vi "Check If Gif Valid.vi"(8 "error in (no error)":errorcluster caption="错误输入（无错误）", 9 "Version":string, 10 "Signature":string, 11 "Gif Image 输入":refnum<class "Gif Image.lvclass"> caption="DNL_LabVIEW Object in") -> (0 "error out":errorcluster caption="错误输出", 2 "Valid":bool, 3 "Gif Image 输出":refnum<class "Gif Image.lvclass"> caption="DNL_LabVIEW Object out")   [LabVIEW 2012, in "Picture Box Tools.lvlib" / "Gif Image.lvclass"]
uses:
  Gif Image.lvclass
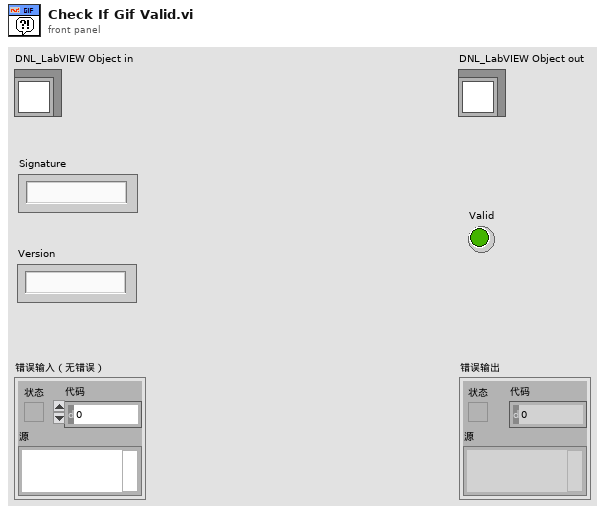
[diagram p1: front panel]
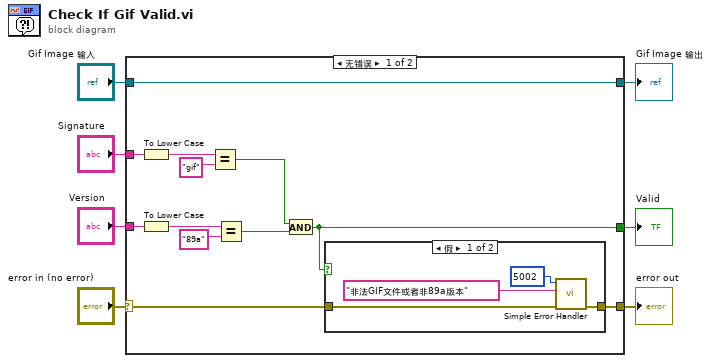
[diagram p0: block diagram]
diagram:
  n1 = case shown="无错误" "error in (no error)" {
    selector: "error in (no error)" -> [w9 w26]
    tunnel: [w8 w26] -> w6
    tunnel: [w19 w25] -> w4
    tunnel: "Gif Image 输入" -> [w19 w25]
    tunnel: "Signature" -> [w18 _]
    tunnel: "Version" -> [w17 _]
    tunnel: [w10 _] -> w1
    frame No Error {
      n2 = To Lower Case(string=w18) -> (all lower case string=w16:string)
      n3 = To Lower Case(string=w17) -> (all lower case string=w14:string)
      n4 = Equal?(x=w16, y="gif") -> (x = y?=w12:bool)
      n5 = Equal?(x=w14, y="89a") -> (x = y?=w11:bool)
      n6 = And(x=w12, y=w11) -> (x .and. y?=w10:bool)
      n7 = case shown="假" w10 {
        tunnel: w9 -> [w21 w24]
        tunnel: [w20 w24] -> w8
        frame False {
          n8 = call <vilib>:"Simple Error Handler.vi"("error code (no error:0)"=5002, "error source (\" \")"="非法GIF文件或者非89a版本" ("error source (\" \")"), "error in (no error)"=w21) -> ("error out"=w20:errorcluster)  [unwired: 2 in, 4 out]
        }
        frame True {
        }
      }
    }
    frame Error {
    }
  }
  "error out" <- w6
  "Gif Image 输出" <- w4
  "Valid" <- w1
